vi "setConfiguration.vi"(8 "error in (no error)":errorcluster, 10 "Configuration":T1, 11 "ExampleInstrument in":refnum<class "Instrument.Template.lvclass">) -> (0 "error out":errorcluster, 3 "ExampleInstrument out":refnum<class "Instrument.Template.lvclass">)   [LabVIEW 2019, in "Instrument.Template.lvclass"]
uses:
  Instrument.Template.lvclass
  SMOs/Instrument/Typedefs/Instrument.Commands--Enum.ctl
  SMOs/Instrument/Instrument.lvclass
  ba1f4714-505f-4f81-9d88-8be6534450d0.vi
  Typedefs/Instrument.Template.Configuration--Cluster.ctl
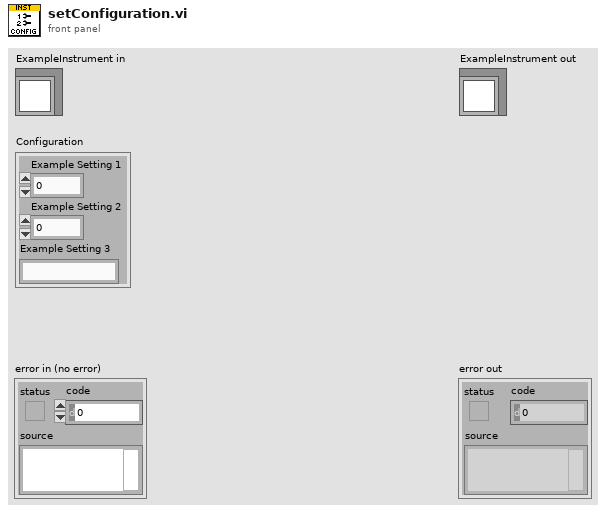
[diagram p1: front panel]
types:
  T1 = typedef "Instrument.Template.lvclass/Instrument.Template.Configuration--Cluster.ctl" = cluster{"Example Setting 1":dbl, "Example Setting 2":dbl, "Example Setting 3":string}
  T2 = typedef "Instrument.lvclass/Instrument.Commands--Enum.ctl" = enum16{"HELP", "ACK", "setConfiguration", "getAll", "getAllData"}
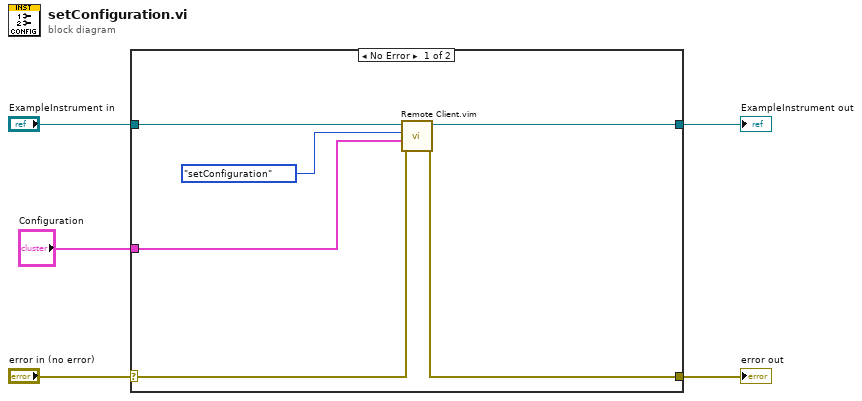
[diagram p0: block diagram]
diagram:
  n1 = case shown="No Error" "error in (no error)" {
    selector: "error in (no error)" -> [w7 w13]
    tunnel: [w6 w13] -> w4
    tunnel: [w8 w12] -> w2
    tunnel: "ExampleInstrument in" -> [w9 w12]
    tunnel: "Configuration" -> [w10 _]
    frame No Error {
      n2 = call "Remote Client.vim"("error in (no error)"=w7, "params"=w10, "method"=Instrument.Commands--Enum."setConfiguration" ("Commands"), "Instrument in"=w9) -> ("error out"=w6:errorcluster, "Instrument out"=w8:refnum<class "Instrument.Template.lvclass">)  [unwired: 4 in, 2 out]
    }
    frame Error {
    }
  }
  "error out" <- w4
  "ExampleInstrument out" <- w2
